vi "Client Single Connection.vi"() -> ()   [LabVIEW 2013]
doc: "This VI acts as a server for an incoming websockets connection. Receives/sends string data to the connected client."
uses:
  WebSockets/WebSocket Client/WebSocket Client.lvclass
  WebSockets/WebSocket/WebSocket.lvclass/WebSocket.ctl
  WebSockets/WebSocket/WebSocket.lvclass
panel:
  in  "Disconnect":bool
  in  "Connect":bool
  in  "WebSockets URL":string="ws://echo.websocket.org"
  out "HTTP Headers":variant
  in  "Stop":bool
  out "Received Data":string
  in  "Send":bool
  in  "Data":string
  # "WebSockets Client Example"
  # "This VI is a simple example of sending/receiving data using WebSockets.\nIt opens a WebSockets Client connection to the WebSockets URL and can send / receive WebSockets data from the server.\n\nInstructions for use:\n1) Run this VI\n2) Enter the WebSockets URL that you wish to open a connection to (e.g. ws://echo.websocket.org) and click 'Connect'\n3) Enter text to send in 'Data' hit 'Send' to send to the WebSockets server\n4) WebSockets messages received from the server will be displayed in 'Received Data'"
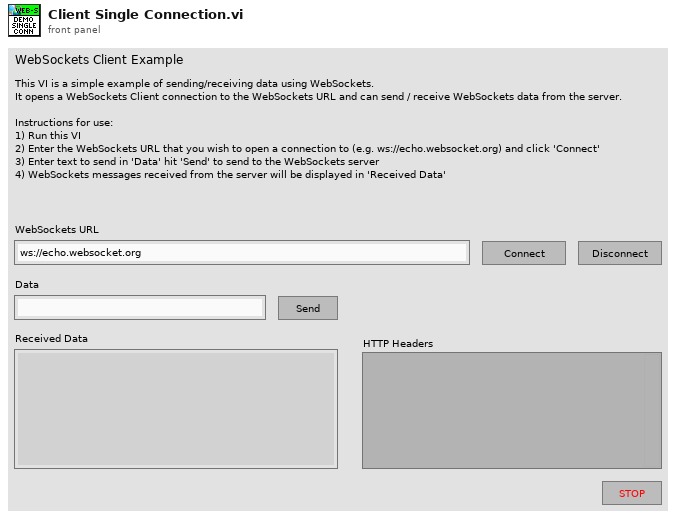
[diagram p1: front panel]
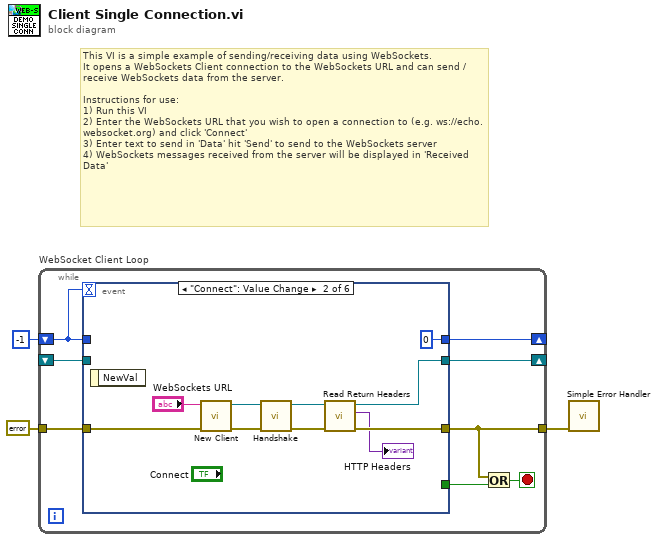
[diagram p0: block diagram]
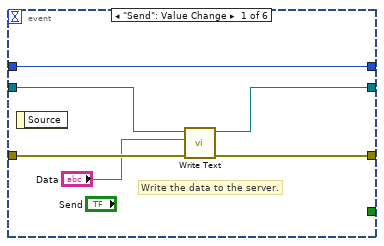
[diagram p2: hidden frame]
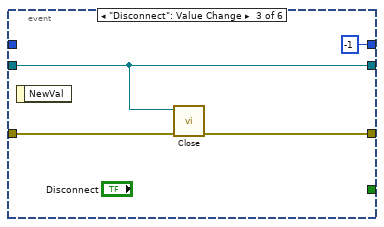
[diagram p3: hidden frame]
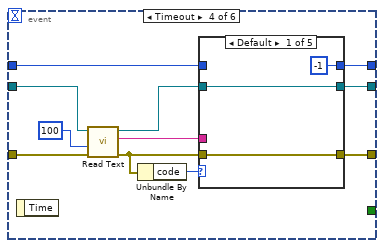
[diagram p4: hidden frame]
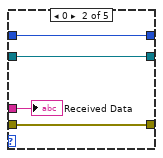
[diagram p5: hidden frame]
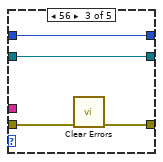
[diagram p6: hidden frame]
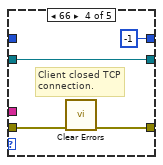
[diagram p7: hidden frame]
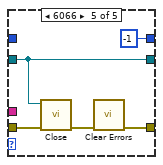
[diagram p8: hidden frame]
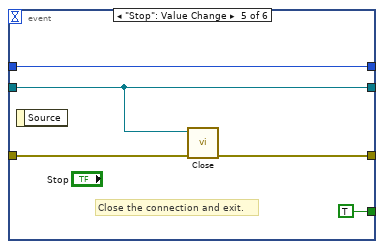
[diagram p9: hidden frame]
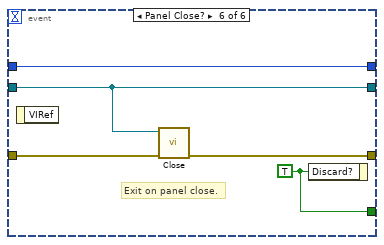
[diagram p10: hidden frame]
diagram:
  # "This VI is a simple example of sending/receiving data using WebSockets.\nIt opens a WebSockets Client connection to the WebSockets URL and can send / receive WebSockets data from the server.\n\nInstructions for use:\n1) Run this VI\n2) Enter the WebSockets URL that you wish to open a connection to (e.g. ws://echo.websocket.org) and click 'Connect'\n3) Enter text to send in 'Data' hit 'Send' to send to the WebSockets server\n4) WebSockets messages received from the server will be displayed in 'Received Data'"
  n1 = while "WebSocket Client Loop" {
    tunnel: [w8] -> w3
    tunnel: errorcluster {"status"=FALSE, "code"=0, "source"=""} ("error out") -> [w11]
    shift-right: [w7] -> _
    shift-left: _ -> [w6]
    shift-right: [w5] -> _
    shift-left: -1 -> [w4]
    stop <- w9 stop-if-true
    n2 = event shown="[1] \"Connect\": Value Change" {
      selector: _ -> [_ _ _ _ _ _]
      dyn-events: _ -> [_ _ _ _ _ _]
      timeout: w4 -> [_ _ _ _ _ _]
      tunnel: [_ _ _ _ TRUE w72] -> w10
      tunnel: [w16 w20 w29 w37 w65 w70] -> w8
      tunnel: w11 -> [w17 w26 w31 w42 w66 w71]
      tunnel: [w13 w21 w30 w34 w64 w69] -> w7
      tunnel: w6 -> [w14 _ w30 w41 w64 w69]
      tunnel: w4 -> [w12 _ _ w33 w63 w68]
      tunnel: [w12 0 -1 w32 w63 w68] -> w5
      event "Send": Value Change {
        # "Write the data to the server."
        n3 = event-data() -> ()  [unwired: 1 in, 1 out]
        n4 = call-dynamic "Write Text.vi"("error in (no error)"=w17, "String Data"="Data", "WebSocket in"=w14) -> ("error out"=w16:errorcluster, "WebSocket out"=w13:refnum<class "WebSocket Client.lvclass">)  [unwired: 7 in]
      }
      event "Connect": Value Change {
        n5 = event-data() -> ()  [unwired: 1 in, 1 out]
        n6 = call "New Client.vi"("error in (no error)"=w26, "WebSocket URL"="WebSockets URL") -> ("error out"=w27:errorcluster, "WebSocket Client out"=w24:refnum<class "WebSocket Client.lvclass">)  [unwired: 8 in]
        n7 = call-dynamic "Handshake.vi"("error in (no error)"=w27, "WebSocket Client in"=w24) -> ("error out"=w23:errorcluster, "WebSocket Client out"=w22:refnum<class "WebSocket Client.lvclass">)  [unwired: 8 in]
        n8 = call "Read Return Headers.vi"("error in (no error)"=w23, "WebSocket in"=w22) -> ("error out"=w20:errorcluster, "Return Headers"=→"HTTP Headers":variant, "WebSocket out"=w21:refnum<class "WebSocket Client.lvclass">)  [unwired: 7 in]
      }
      event "Disconnect": Value Change {
        n9 = event-data() -> ()  [unwired: 1 in, 1 out]
        n10 = call-dynamic "Close.vi"("error in (no error)"=w31, "WebSocket in"=w30) -> ("error out"=w29:errorcluster)  [unwired: 9 in]
      }
      event Timeout {
        n11 = event-data() -> ()  [unwired: 1 in, 1 out]
        n12 = call-dynamic "Read Text.vi"("error in (no error)"=w42, "timeout ms (5000)"=100, "WebSocket in"=w41) -> ("error out"=w36:errorcluster, "Data"=w39:string, "WebSocket out"=w35:refnum<class "WebSocket Client.lvclass">)  [unwired: 6 in]
        n13 = Unbundle By Name(w36) -> ("code"=w38:i32)
        n14 = case shown="Default" w38 {
          tunnel: w39 -> [_ w49 _ _ _]
          tunnel: [w45 w48 w52 w54 w58] -> w37
          tunnel: w36 -> [w45 w48 w53 w57 w62]
          tunnel: w35 -> [w44 w47 w51 w56 w60]
          tunnel: [w44 w47 w51 w56 w60] -> w34
          tunnel: w33 -> [_ w46 w50 _ _]
          tunnel: [-1 w46 w50 -1 -1] -> w32
          frame Default {
          }
          frame 0 {
            "Received Data" <- w49
          }
          frame 56 {
            n15 = call <vilib>:"Clear Errors.vi"("error in (no error)"=w53) -> ("error out"=w52:errorcluster)  [unwired: 6 in]
          }
          frame 66 {
            # "Client closed TCP connection."
            n16 = call <vilib>:"Clear Errors.vi"("error in (no error)"=w57) -> ("error out"=w54:errorcluster)  [unwired: 6 in]
          }
          frame 6066 {
            n17 = call-dynamic "Close.vi"("error in (no error)"=w62, "WebSocket in"=w60) -> ("error out"=w61:errorcluster)  [unwired: 9 in]
            n18 = call <vilib>:"Clear Errors.vi"("error in (no error)"=w61) -> ("error out"=w58:errorcluster)  [unwired: 6 in]
          }
        }
      }
      event "Stop": Value Change {
        # "Close the connection and exit."
        n19 = event-data() -> ()  [unwired: 1 in, 1 out]
        n20 = call-dynamic "Close.vi"("error in (no error)"=w66, "WebSocket in"=w64) -> ("error out"=w65:errorcluster)  [unwired: 9 in]
      }
      event Panel Close? {
        w72 = TRUE ("Discard?")
        # "Exit on panel close."
        n21 = event-data() -> ()  [unwired: 1 in, 1 out]
        n22 = call-dynamic "Close.vi"("error in (no error)"=w71, "WebSocket in"=w69) -> ("error out"=w70:errorcluster)  [unwired: 9 in]
        n23 = event-data("Discard?"=w72) -> ()  [unwired: 1 in, 1 out]
      }
    }
    n24 = Or(x=w8, y=w10) -> (x .or. y?=w9:bool)
  }
  n25 = call <vilib>:"Simple Error Handler.vi"("error in (no error)"=w3) -> ()  [unwired: 4 in, 5 out]
